vi "HEX整型数正则表达式（精确整型数，字符串）.vi"(8 "error in (no error)":errorcluster caption="错误输入（无错误）", 11 "位数":i32) -> (0 "error out":errorcluster caption="错误输出", 3 "正则表达式":string)   [LabVIEW 2011]
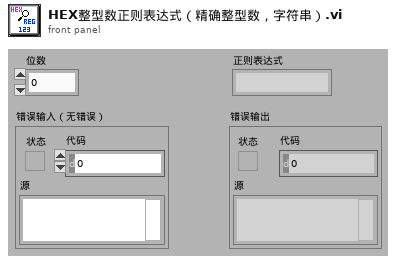
[diagram p1: front panel]
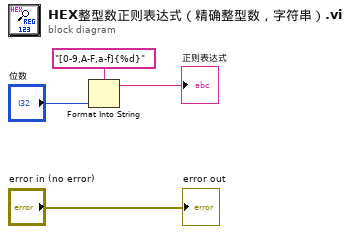
[diagram p0: block diagram]
diagram:
  n1 = Format Into String(format string="[0-9,A-F,a-f]{%d}" ("格式字符串"), "位数") -> (resulting string=→"正则表达式":string)  [unwired: 2 in, 1 out]
  "error out" <- "error in (no error)"
